vi "GetSubarrayOfCircularBuffer-Numbers.vi"(8 "buffer":dbl[](array[numeric]), 10 "subset size":i32, 11 "start index":i32) -> (2 "subarray":dbl[](array[numeric]))   [LabVIEW 2016]
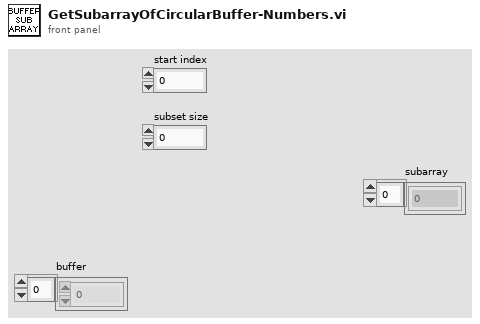
[diagram p1: front panel]
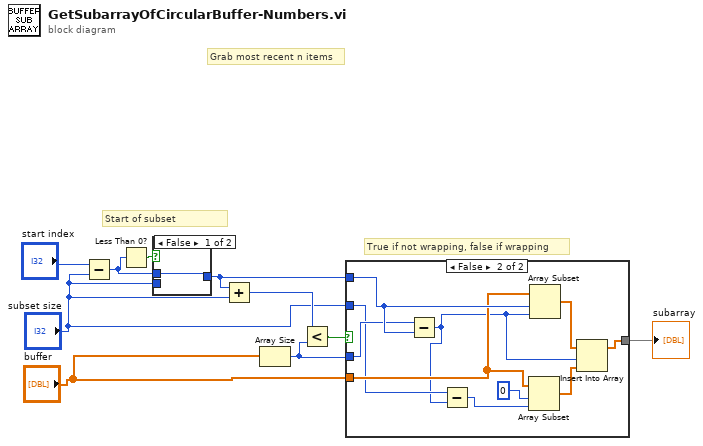
[diagram p0: block diagram]
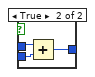
[diagram p2: hidden frame]
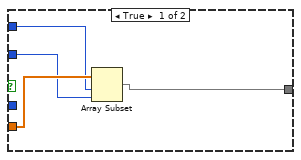
[diagram p3: hidden frame]
diagram:
  # "Start of subset"
  # "Grab most recent n items"
  # "True if not wrapping, false if wrapping"
  n1 = Subtract(x="start index", y="subset size") -> (x-y=w6:i32)
  n2 = Less Than 0?(x=w6) -> (x < 0?=w7:bool)
  n3 = case shown="False" w7 {
    tunnel: w6 -> [w11 w13]
    tunnel: "subset size" -> [_ w14]
    tunnel: [w11 w12] -> w5
    frame False {
    }
    frame True {
      n4 = Add(x=w13, y=w14) -> (x+y=w12:i32)
    }
  }
  n5 = Add(x=w5, y="subset size") -> (x+y=w9:i32)
  n6 = Array Size(array="buffer") -> (size(s)=w3:i32)
  n7 = Less?(x=w9, y=w3) -> (x < y?=w10:bool)
  n8 = case shown="False" w10 {
    tunnel: "buffer" -> [w18 w26]
    tunnel: w5 -> [w17 w28]
    tunnel: "subset size" -> [w16 w24]
    tunnel: w3 -> [_ w27]
    tunnel: [w15 w19] -> w4
    frame True {
      n9 = Array Subset(array=w18, index=w17, length=w16) -> (w15:dbl[])
    }
    frame False, Default {
      n10 = Subtract(x=w27, y=w28) -> (x-y=w21:i32)
      n11 = Subtract(x=w24, y=w21) -> (x-y=w23:i32)
      n12 = Array Subset(array=w26, index=0, length=w23) -> (w20:dbl[])
      n13 = Array Subset(array=w26, index=w28, length=w21) -> (w22:dbl[])
      n14 = Insert Into Array(array=w22, index=w21, new element=w20) -> (w19:dbl[])
    }
  }
  "subarray" <- w4
